vi "Autocomplete popup.vi"(8 "error in (no error)":errorcluster, 11 "input":T1={"Screen Coordinates"={"Horizontal"=0, "Vertical"=0}, "Width"=0, "max rows"=8, "List"=[], "init value"=""}) -> (0 "error out":errorcluster, 2 "Accept?":bool, 3 "String":string)   [LabVIEW 2021, in "Autocomplete popup.lvlib"]
uses:
  Autocomplete popup.lvlib
  subvis/input options.ctl
  <vilib>/Utility/miscctls.llb/LVPointTypeDef.ctl
  Autocomplete Textbox/SubVIs/Loop Data.ctl
  Autocomplete Textbox/SubVIs/Inputs.ctl
  Autocomplete Textbox/Classes/Handle/Listbox placement.ctl
  Autocomplete Textbox/SubVIs/Color String Options.ctl
  Autocomplete Textbox/SubVIs/Refs.ctl
  Autocomplete Textbox/SubVIs/State data.ctl
  <vilib>/Utility/miscctls.llb/LVSelectionTypeDef.ctl
  Autocomplete Textbox/Autocomplete Textbox.lvlib
  Autocomplete Textbox/Classes/Handle/Handle.lvclass
panel:
  in  "String":string
  in  "Listbox":i32(listbox)
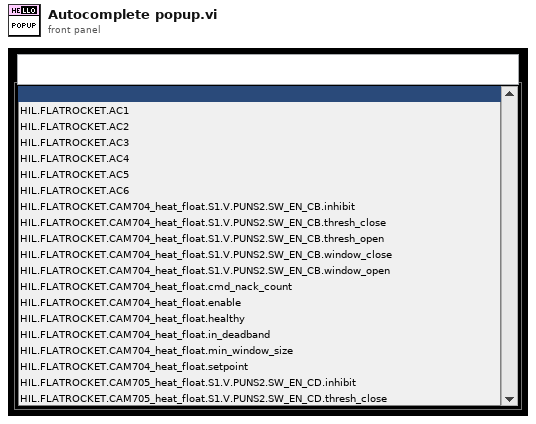
[diagram p1: front panel]
types:
  T1 = typedef "Autocomplete popup.lvlib/input options.ctl" = cluster{"Screen Coordinates":T2, "Width":u32, "max rows":i32, "List":string[], "init value":string}
  T2 = typedef "LVPointTypeDef.ctl" = cluster{"Horizontal":i16, "Vertical":i16}
  T3 = typedef "LVSelectionTypeDef.ctl" = cluster{"Selection Start":u32, "Selection End":u32}
  T4 = typedef "Autocomplete Textbox.lvlib/Handle.lvclass/Listbox placement.ctl" = enum16{"None", "Under String", "Fit to Pane"}
  T5 = typedef "Autocomplete Textbox.lvlib/Inputs.ctl" = cluster{"List":string[], "max rows":i32, "Listbox placement":T4, "String Color Options":T6}
  T6 = typedef "Autocomplete Textbox.lvlib/Color String Options.ctl" = cluster{"Use? (F)":bool, "Color - Valid":u32, "Color - Invalid":u32, "Allow blank?":bool}
  T7 = typedef "Autocomplete Textbox.lvlib/Loop Data.ctl" = cluster{"Config":T5, "Refs":T8, "State":T9}
  T8 = typedef "Autocomplete Textbox.lvlib/Refs.ctl" = cluster{"String":refnum<vi>, "Listbox":refnum<vi>}
  T9 = typedef "Autocomplete Textbox.lvlib/State data.ctl" = cluster{"LB active?":bool}
  T10 = enum32{"Invalid", "Standard", "Closed", "Hidden", "Minimized", "Maximized"}
  T11 = typedef "LVRectTypeDef.ctl" = cluster{"Left":i16, "Top":i16, "Right":i16, "Bottom":i16}
  T12 = typedef "eventvkey.ctl" = enum16{"ASCII", "Enter", "Return", "Shift", "Ctrl", "Alt", "Cmd", "Opt", "Caps", "NumLock", "Clear", "Break", "Up", "Down", "Left", "Right", "Insert", "Delete", "Home", "End", "PageUp", "PageDown", "Escape", "Help", "Pause", "ScrollLock", "F1", "F2", "F3", "F4", "F5", "F6", "F7", "F8", "F9", "F10", "F11", "F12", "F13", "F14", "F15", "F16", "F17", "F18", "F19", "F20", "F21", "F22", "F23", "F24", "Play", "VolumeUp", "VolumeDown", "Mute", "Two Byte Char"}
  T13 = typedef "LVPoint32TypeDef.ctl" = cluster{"Horizontal":i32, "Vertical":i32}
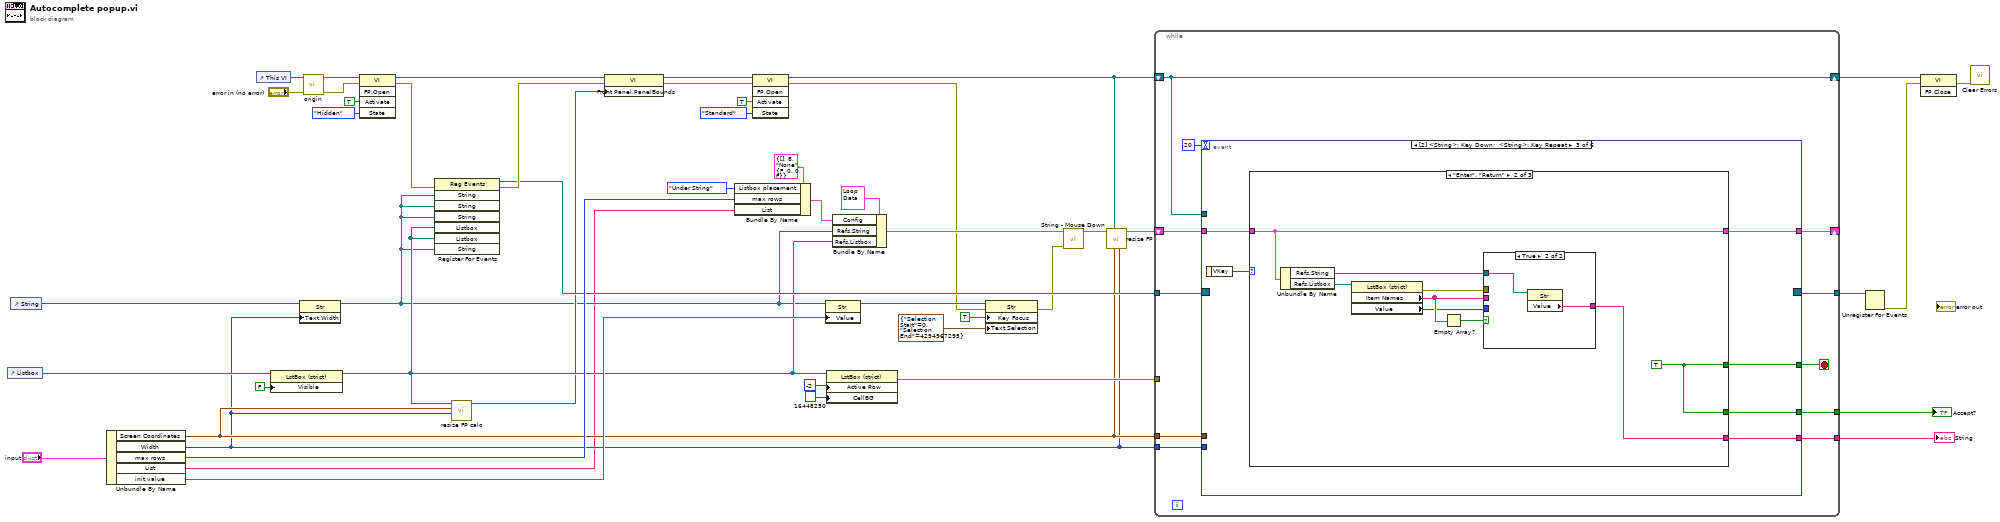
[diagram p0: block diagram]
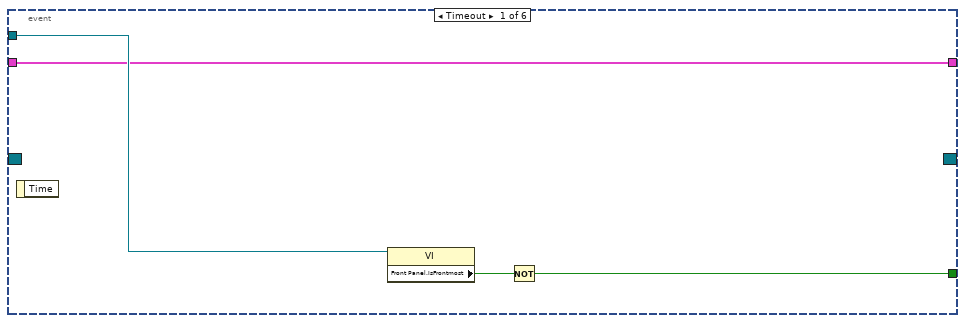
[diagram p2: hidden frame]
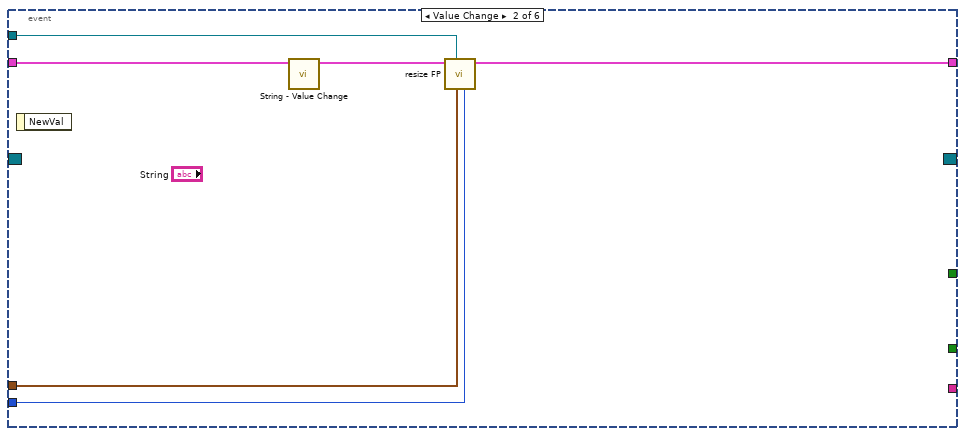
[diagram p3: hidden frame]
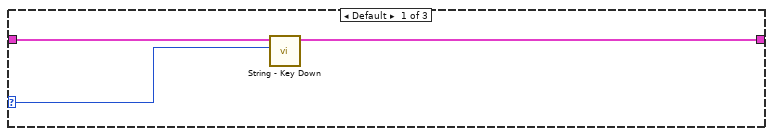
[diagram p4: hidden frame]
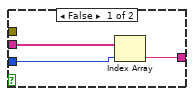
[diagram p5: hidden frame]
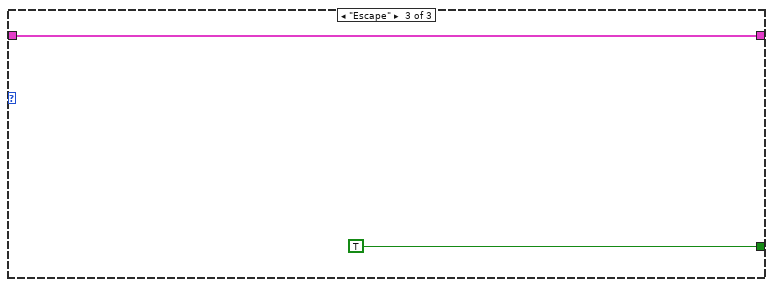
[diagram p6: hidden frame]
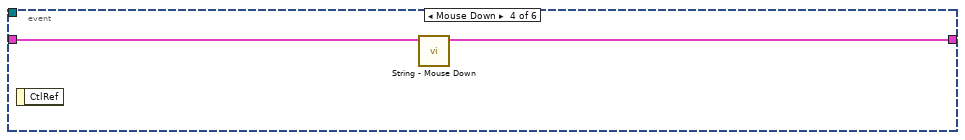
[diagram p7: hidden frame]
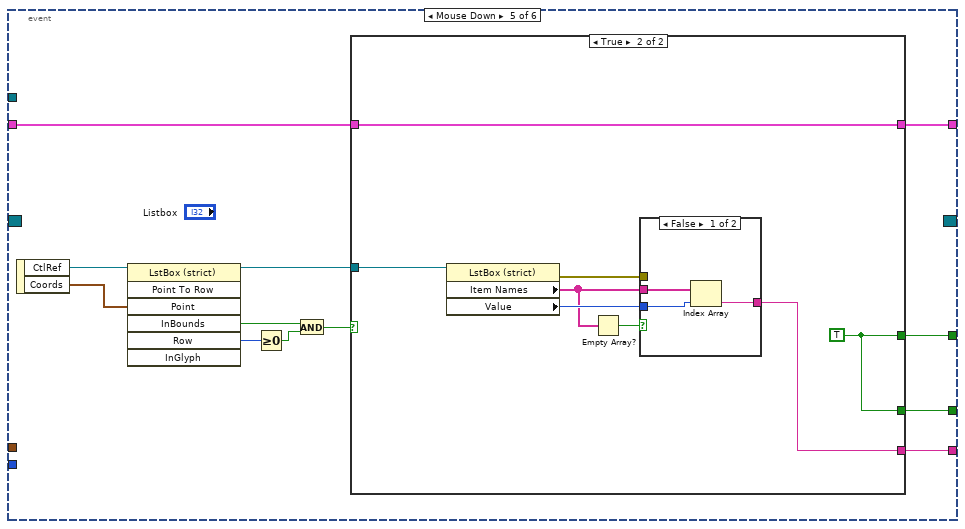
[diagram p8: hidden frame]
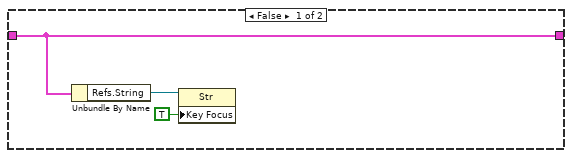
[diagram p9: hidden frame]
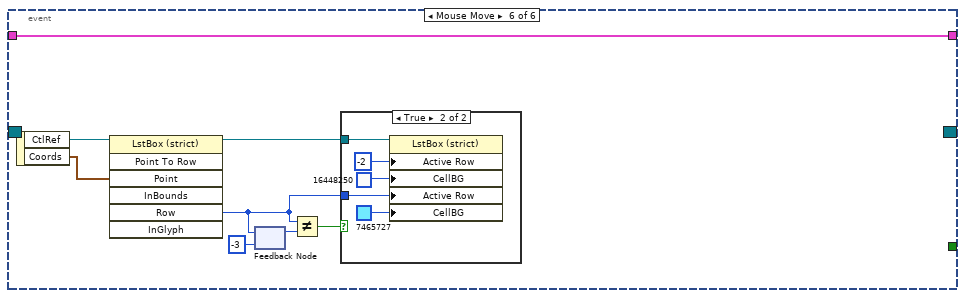
[diagram p11: hidden frame]
diagram:
  n1 = control-ref of="Listbox"() -> (w11:refnum<vi>)
  n2 = control-ref of="String"() -> (w18:refnum<vi>)
  n3 = Unbundle By Name("input") -> ("Screen Coordinates"=w5:T2, "Width"=w4:u32, "max rows"=w33:i32, "List"=w1:string[], "init value"=w30:string)
  n4 = control-ref of="This VI"() -> (w27:refnum<vi>)
  n5 = property class="LstBox (strict)"(reference=w11, "Visible"=FALSE) -> (reference out=w10:refnum<vi>)  [unwired: 1 in, 1 out]
  n6 = property class="Str"(reference=w18, "Text.Width"=w4) -> (reference out=w3:refnum<vi>)  [unwired: 1 in, 1 out]
  n7 = call "origin.vi"("error in (no error)"="error in (no error)", "vi ref"=w27) -> ("error out"=w24:errorcluster, "vi ref"=w25:refnum<vi>)  [unwired: 8 in]
  n8 = invoke class="VI" method="FP.Open"(reference=w25, error in=w24, "Activate"=TRUE ("Activate?"), "State"=T10."Hidden") -> (reference out=w46:refnum<vi>, error out=w36:errorcluster)  [unwired: 1 in, 3 out]
  n9 = register-events(error in=w36, w3, w3, w3, w10, w10, w3) -> (reference out=w31:refnum<event-registration>, error out=w35:errorcluster)  [unwired: 1 in]
  n10 = call "resize FP calc.vi"("Width"=w4, "Screen Coordinates"=w5, "refs.listbox"=w10) -> ("fp bounds"=w9:T11)  [unwired: 8 in]
  n11 = property class="VI"(reference=w46, error in=w35, "Front Panel.PanelBounds"=w9) -> (reference out=w43:refnum<vi>, error out=w42:errorcluster)
  n12 = Bundle By Name(cluster=T5 {"List"=[], "max rows"=8, "Listbox placement"=enum."None", "String Color Options"={"Use? (F)"=FALSE, "Color - Valid"=0, "Color - Invalid"=0, "Allow blank?"=FALSE}} ("Config"), "Listbox placement"=Listbox_placement."Under String", "max rows"=w33, "List"=w1) -> (w40:T5)
  n13 = invoke class="VI" method="FP.Open"(reference=w43, error in=w42, "Activate"=TRUE ("Activate?"), "State"=T10."Standard") -> (reference out=w6:refnum<vi>, error out=w21:errorcluster)  [unwired: 1 in, 3 out]
  n14 = property class="Str"(reference=w3, "Value"=w30) -> (reference out=w22:refnum<vi>)  [unwired: 1 in, 1 out]
  n15 = property class="LstBox (strict)"(reference=w10, "Active Row"=-2 ("Active Row:Active Row Number"), "CellBG"=u32 16448250) -> (error out=w37:errorcluster)  [unwired: 1 in, 1 out]
  n16 = Bundle By Name(cluster=T7 {"Config"={"List"=[], "max rows"=8, "Listbox placement"=enum."None", "String Color Options"={"Use? (F)"=FALSE, "Color - Valid"=0, "Color - Invalid"=0, "Allow blank?"=FALSE}}, "Refs"={"String"=refnum, "Listbox"=refnum}, "State"={"LB active?"=FALSE}} ("Cluster"), "Config"=w40, "Refs.String"=w3, "Refs.Listbox"=w10) -> (w23:T7)
  n17 = property class="Str"(reference=w22, error in=w21, "Key Focus"=TRUE, "Text.Selection"=T3 {"Selection Start"=0, "Selection End"=4294967295}) -> (error out=w16:errorcluster)  [unwired: 1 out]
  n18 = call "String - Mouse Down.vi"("error in (no error)"=w16, "Loop data in"=w23) -> ("Loop data out"=w8:T7)  [unwired: 8 in, 1 out]
  n19 = call "resize FP.vi"("Width"=w4, "Screen Coordinates"=w5, "vi ref"=w6, "Loop data in"=w8) -> ("Loop data out"=w7:T7)  [unwired: 6 in, 1 out]
  n20 = while {
    tunnel: w31 -> [w59]
    shift-right: [w58] -> _
    shift-left: w7 -> [w56]
    tunnel: w37 -> [_]
    shift-right: [w54] -> w28
    shift-left: w6 -> [w54]
    tunnel: [w53] -> w20
    tunnel: [w52] -> w15
    tunnel: [w51] -> w14
    tunnel: w5 -> [w50]
    tunnel: w4 -> [w49]
    stop <- w57 stop-if-true
    n21 = event shown="[2] <String>: Key Down;  <String>: Key Repeat" {
      selector: w59 -> [_ _ _ _ _ _]
      dyn-events: [_ _ _ _ _ _] -> w53
      timeout: 20 -> [_ _ _ _ _ _]
      tunnel: w56 -> [w62 w69 w73 w96 w102 w123]
      tunnel: [w62 w67 w72 w95 w101 w123] -> w58
      tunnel: [w60 _ w74 _ w100 _] -> w57
      tunnel: w54 -> [w63 w66 _ _ _ _]
      tunnel: [_ _ w71 _ w99 _] -> w52
      tunnel: [_ _ w70 _ w97 _] -> w51
      tunnel: w50 -> [_ w65 _ _ _ _]
      tunnel: w49 -> [_ w64 _ _ _ _]
      event Timeout {
        n22 = event-data() -> ()  [unwired: 1 in, 1 out]
        n23 = property class="VI"(reference=w63) -> ("Front Panel.IsFrontmost"=w61:bool)  [unwired: 1 in, 2 out]
        n24 = Not(x=w61) -> (.not. x?=w60:bool)
      }
      event Value Change {
        n25 = event-data() -> ()  [unwired: 1 in, 1 out]
        n26 = call "String - Value Change.vi"("Loop data in"=w69) -> ("Loop data out"=w68:T7)  [unwired: 9 in, 1 out]
        n27 = call "resize FP.vi"("Width"=w64, "Screen Coordinates"=w65, "vi ref"=w66, "Loop data in"=w68) -> ("Loop data out"=w67:T7)  [unwired: 6 in, 1 out]
      }
      event Key Down; Key Repeat {
        n28 = event-data() -> ("VKey"=w75:T12)  [unwired: 1 in]
        n29 = case shown="\"Enter\", \"Return\"" w75 {
          selector: w75 -> [w76 _ _]
          tunnel: [_ w87 TRUE] -> w74
          tunnel: w73 -> [w78 w81 w93]
          tunnel: [w77 w81 w93] -> w72
          tunnel: [_ w87 _] -> w71
          tunnel: [_ w80 _] -> w70
          frame Default {
            n30 = call "String - Key Down.vi"("VKey"=w76, "Loop data in"=w78) -> ("Loop data out"=w77:T7)  [unwired: 8 in, 1 out]
          }
          frame "Enter", "Return" {
            w87 = TRUE
            n31 = Unbundle By Name(w81) -> ("Refs.String"=w79:refnum<vi>, "Refs.Listbox"=w83:refnum<vi>)
            n32 = property class="LstBox (strict)"(reference=w83) -> (error out=w84:errorcluster, "Item Names"=w85:string[], "Value"=w82:i32)  [unwired: 1 in, 1 out]
            n33 = Empty Array?(array=w85) -> (empty?=w86:bool)
            n34 = case shown="True" w86 {
              tunnel: w82 -> [w90 _]
              tunnel: w84 -> [_ _]
              tunnel: w85 -> [w89 _]
              tunnel: [w88 w91] -> w80
              tunnel: w79 -> [_ w92]
              frame False {
                n35 = Index Array(array=w89, index=w90) -> (element=w88:string)
              }
              frame True {
                n36 = property class="Str"(reference=w92) -> ("Value"=w91:string)  [unwired: 1 in, 2 out]
              }
            }
          }
          frame "Escape" {
          }
        }
      }
      event Mouse Down {
        n37 = event-data() -> ()  [unwired: 1 in, 1 out]
        n38 = call "String - Mouse Down.vi"("Loop data in"=w96) -> ("Loop data out"=w95:T7)  [unwired: 9 in, 1 out]
      }
      event Mouse Down {
        n39 = event-data() -> ("CtlRef"=w108:refnum<vi>, "Coords"=w107:T13)  [unwired: 1 in]
        n40 = invoke class="LstBox (strict)" method="Point To Row"(reference=w108, "Point"=w107) -> (reference out=w98:refnum<vi>, "InBounds"=w105:bool, "Row"=w106:i32)  [unwired: 5 in, 4 out]
        n41 = Greater Or Equal To 0?(x=w106) -> (x >= 0?=w104:bool)
        n42 = And(x=w105, y=w104) -> (x .and. y?=w103:bool)
        n43 = case shown="True" w103 {
          tunnel: w102 -> [w109 w118]
          tunnel: [w109 w118] -> w101
          tunnel: [_ w119] -> w100
          tunnel: [_ w119] -> w99
          tunnel: w98 -> [_ w113]
          tunnel: [_ w112] -> w97
          frame False {
            n44 = Unbundle By Name(w109) -> ("Refs.String"=w110:refnum<vi>)
            n45 = property on="Property Node" class="Str"(reference=w110, "Key Focus"=TRUE) -> ()  [unwired: 1 in, 2 out]
          }
          frame True {
            w119 = TRUE
            n46 = property class="LstBox (strict)"(reference=w113) -> (error out=w116:errorcluster, "Item Names"=w115:string[], "Value"=w117:i32)  [unwired: 1 in, 1 out]
            n47 = Empty Array?(array=w115) -> (empty?=w114:bool)
            n48 = case shown="False" w114 {
              tunnel: w117 -> [w122 _]
              tunnel: w116 -> [_ _]
              tunnel: w115 -> [w121 _]
              tunnel: [w120 _] -> w112
              frame False {
                n49 = Index Array(array=w121, index=w122) -> (element=w120:string)
              }
              frame True {
              }
            }
          }
        }
      }
      event Mouse Move {
        n50 = event-data() -> ("CtlRef"=w125:refnum<vi>, "Coords"=w124:T13)  [unwired: 1 in]
        n51 = invoke class="LstBox (strict)" method="Point To Row"(reference=w125, "Point"=w124) -> (reference out=w130:refnum<vi>, "Row"=w127:i32)  [unwired: 5 in, 5 out]
        n52 = feedback #1(-3 ("Row")) -> (w128:i32)
        n53 = feedback-in #1(w127) -> ()
        n54 = Not Equal?(x=w127, y=w128) -> (x != y?=w126:bool)
        n55 = case shown="True" w126 {
          tunnel: w130 -> [_ w132]
          tunnel: w127 -> [_ w131]
          frame False {
          }
          frame True {
            n56 = property class="LstBox (strict)"(reference=w132, "Active Row"=-2 ("Active Row:Active Row Number"), "CellBG"=u32 16448250, "Active Row"=w131, "CellBG"=u32 7465727) -> ()  [unwired: 1 in, 2 out]
          }
        }
      }
    }
  }
  "Accept?" <- w15
  "String" <- w14
  n57 = Unregister For Events(event registration refnum=w20) -> (error out=w19:errorcluster)  [unwired: 1 in]
  n58 = invoke class="VI" method="FP.Close"(reference=w28, error in=w19) -> (error out=w29:errorcluster)  [unwired: 1 in, 2 out]
  n59 = call <vilib>:"Clear Errors.vi"("error in (no error)"=w29) -> ()  [unwired: 5 in, 2 out]
